vi "FGV Map Get Data (String).vi"(8 "error in (no error)":errorcluster, 10 "Data Key":string, 11 "Instance Key":string) -> (0 "error out":errorcluster, 2 "Data Not Found ?":bool, 3 "Data Out":string)   [LabVIEW 2020, in "FGV Map.lvlib"]
uses:
  FGV Map.lvlib
  Controls/FGV Map Core State.ctl
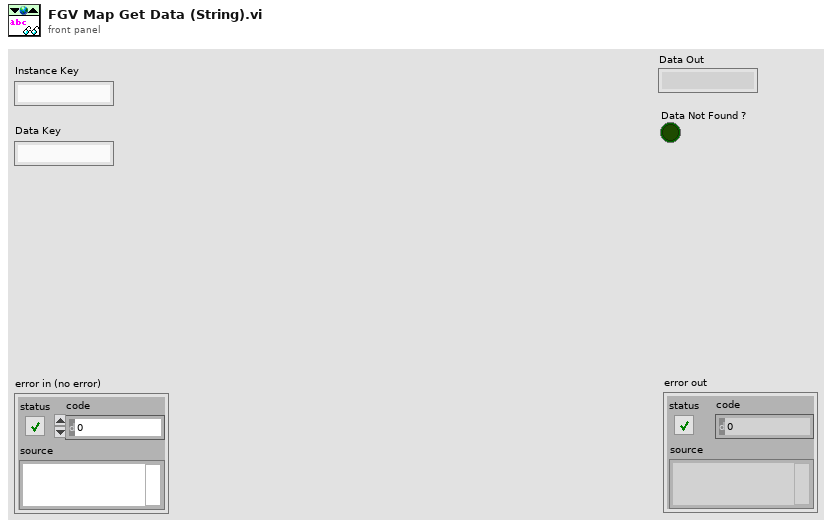
[diagram p1: front panel]
types:
  T1 = typedef "FGV Map.lvlib/FGV Map Core State.ctl" = enum16{"Init", "Set Instance (Unlock)", "Get Instance", "Get Instance (Lock)", "Unlock", "Get All Instances", "Delete Instance"}
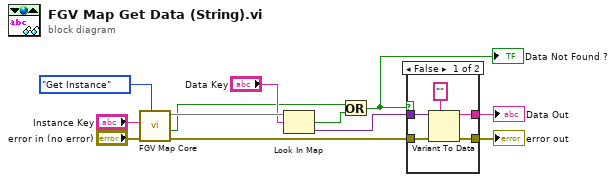
[diagram p0: block diagram]
diagram:
  n1 = call "FGV Map Core.vi"("FGV State"=FGV_Map_Core_State."Get Instance", "error in"="error in (no error)", "Instance Key"="Instance Key") -> ("error out"=w5:errorcluster, "Instance Not Found ?"=w8:bool, "Instance Out"=w10:map{string, variant})  [unwired: 4 in, 2 out]
  n2 = Look In Map(map=w10, key="Data Key") -> (key not found?=w7:bool, value=w4:variant)  [unwired: 1 in]
  n3 = Or(x=w8, y=w7) -> (x .or. y?=w1:bool)
  "Data Not Found ?" <- w1
  n4 = case shown="False" w1 {
    tunnel: w5 -> [w17 w18]
    tunnel: w4 -> [w16 _]
    tunnel: [w14 _] -> w3
    tunnel: [w13 w18] -> w2
    frame False {
      n5 = Variant To Data(error in=w17, type="", Variant=w16) -> (data=w14:string, error out=w13:errorcluster)
    }
    frame True {
    }
  }
  "error out" <- w2
  "Data Out" <- w3
